vi "Unbundle.vi"(10 "index":i32, 11 "[Data Out]":T1[](array[typedef])) -> (0 "State 3":bool, 1 "State 2":bool, 2 "State 1":bool, 3 "Numeric":dbl)   [LabVIEW 2020]
doc: "This subVI receives an array of clusters and extract its individual values."
uses:
  Controls/CLD 6 CSV file data structure.ctl
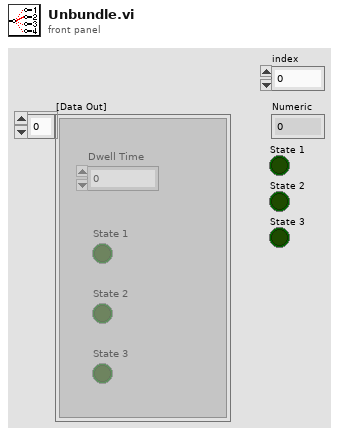
[diagram p1: front panel]
types:
  T1 = typedef "CLD 6 CSV file data structure.ctl" = cluster{"Dwell Time":i32, "State 1":bool, "State 2":bool, "State 3":bool}
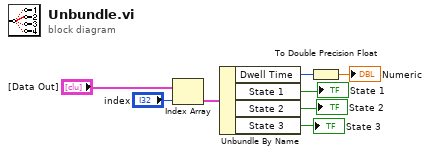
[diagram p0: block diagram]
diagram:
  n1 = Index Array(array="[Data Out]", index="index") -> (element=w6:T1)
  n2 = Unbundle By Name(w6) -> ("Dwell Time"=w8:i32, "State 1"=→"State 1":bool, "State 2"=→"State 2":bool, "State 3"=→"State 3":bool)
  n3 = To Double Precision Float(number=w8) -> (double precision float=→"Numeric":dbl)
